vi "1 - 测试机台交互.vi"(6 "测试机台选择":tag="VB8012-30F490B", 7 "Error In":errorcluster caption="Error In (no error)", 8 "逻辑分析仪参数输入":T2, 9 "可编程电源参数输入":T3, 10 "显示控件引用输入":T1) -> (0 "error out":errorcluster caption="错误输出", 2 "采集信号输出":waveform(dbl)[](array[waveform]), 3 "显示控件引用输出":T1)   [LabVIEW 2019]
uses:
  <vilib>/VirtualBench/_PS Configure Voltage Output0.vi
  <vilib>/VirtualBench/_FGEN Configure Standard Waveform0.vi
  <vilib>/VirtualBench/_MSO Configure Timing0.vi
  <vilib>/VirtualBench/_MSO Configure Digital Edge Trigger0.vi
  <vilib>/VirtualBench/_MSO Configure Analog Edge Trigger0.vi
  <vilib>/VirtualBench/_MSO Configure Digital Pattern Trigger0.vi
  <vilib>/VirtualBench/VirtualBench.lvlib
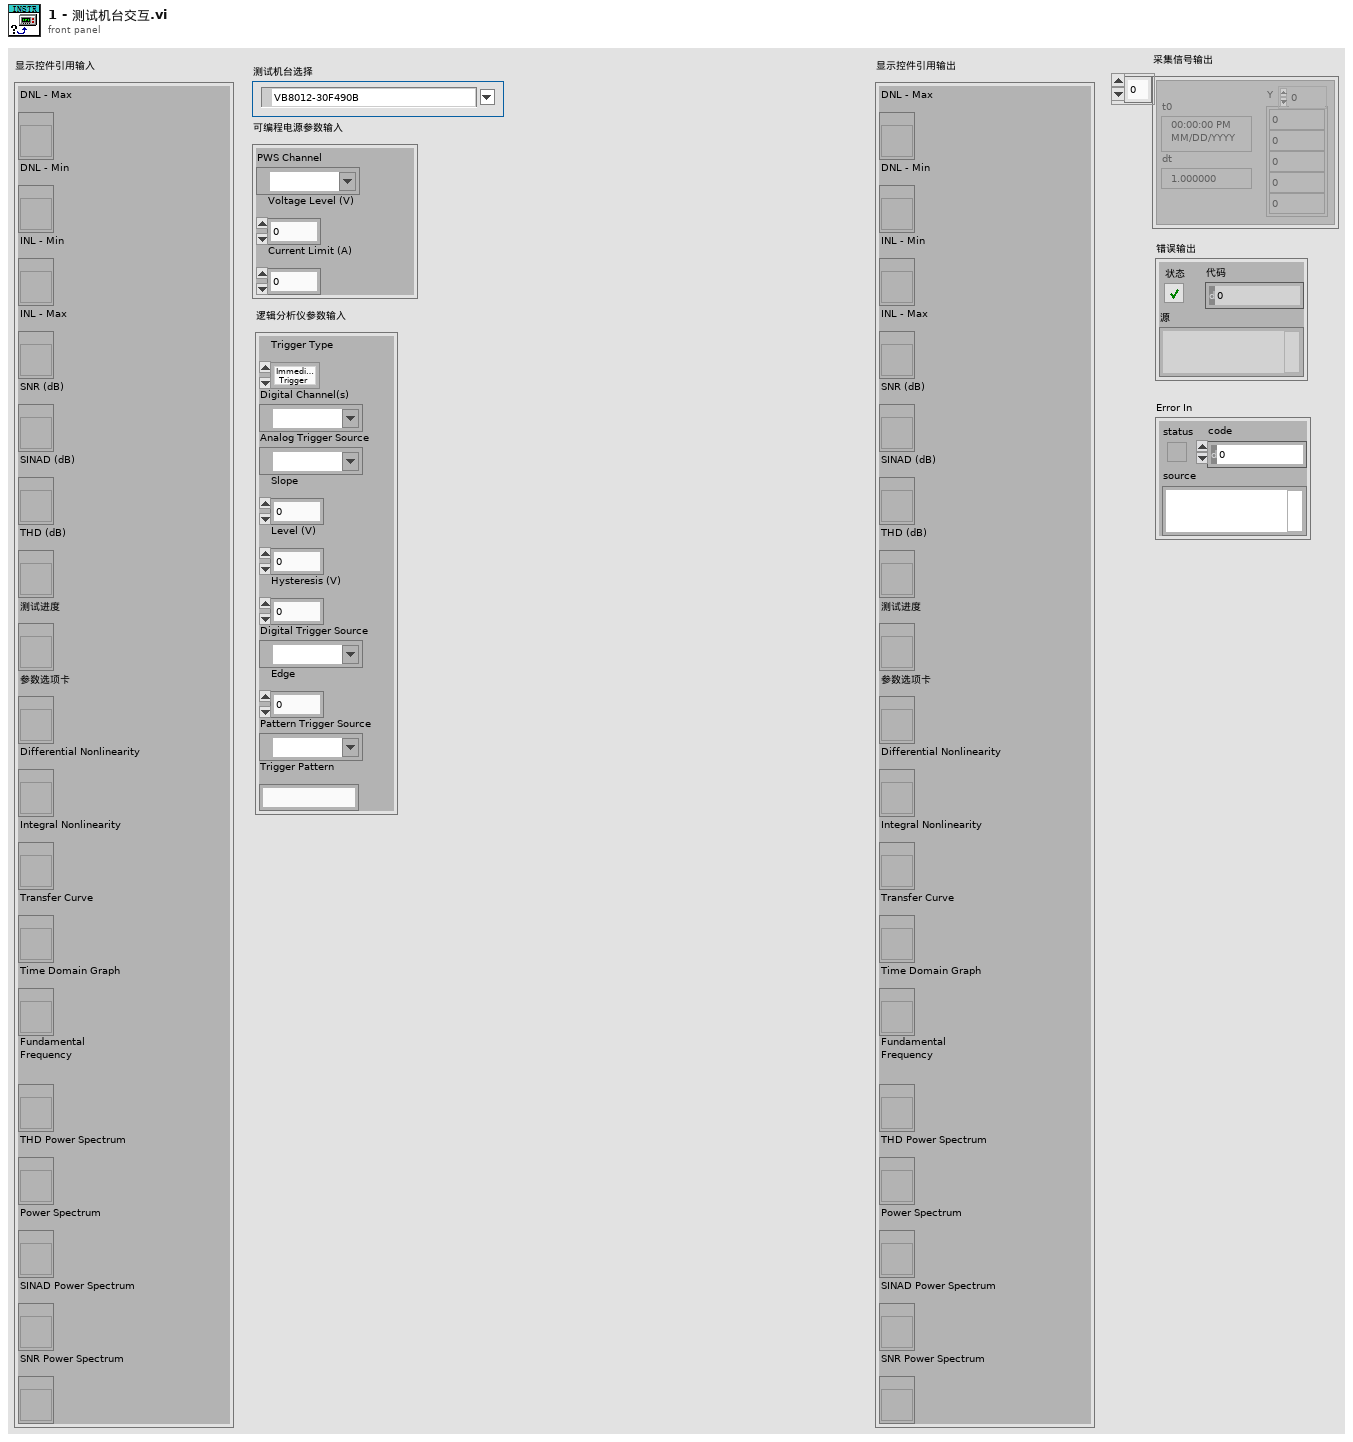
[diagram p1: front panel]
types:
  T1 = cluster{"DNL - Max":refnum<vi>, "DNL - Min":refnum<vi>, "INL - Min":refnum<vi>, "INL - Max":refnum<vi>, "SNR (dB)":refnum<vi>, "SINAD (dB)":refnum<vi>, "THD (dB)":refnum<vi>, "测试进度":refnum<vi>, "参数选项卡":refnum<vi>, "Differential Nonlinearity":refnum<vi>, "Integral Nonlinearity":refnum<vi>, "Transfer Curve":refnum<vi>, "Time Domain Graph":refnum<vi>, "Fundamental\nFrequency":refnum<vi>, "THD Power Spectrum":refnum<vi>, "Power Spectrum":refnum<vi>, "SINAD Power Spectrum":refnum<vi>, "SNR Power Spectrum":refnum<vi>}
  T2 = cluster{"Trigger Type":enum32{"Immediate Trigger", "Digital Trigger", "Analog Trigger", "Pattern Trigger"}, "Digital Channel(s)":tag, "Analog Trigger Source":tag, "Slope":i32, "Level (V)":dbl, "Hysteresis (V)":dbl, "Digital Trigger Source":tag, "Edge":i32, "Pattern Trigger Source":tag, "Trigger Pattern":string}
  T3 = cluster{"PWS Channel":tag, "Voltage Level (V)":dbl, "Current Limit (A)":dbl}
  T4 = enum32{"Time Domain", "Power Spectrum", "THD", "SINAD", "SNR", "DNL", "INL", "Transfer Curve"}
  T5 = enum32{"Immediate Trigger", "Digital Trigger", "Analog Trigger", "Pattern Trigger"}
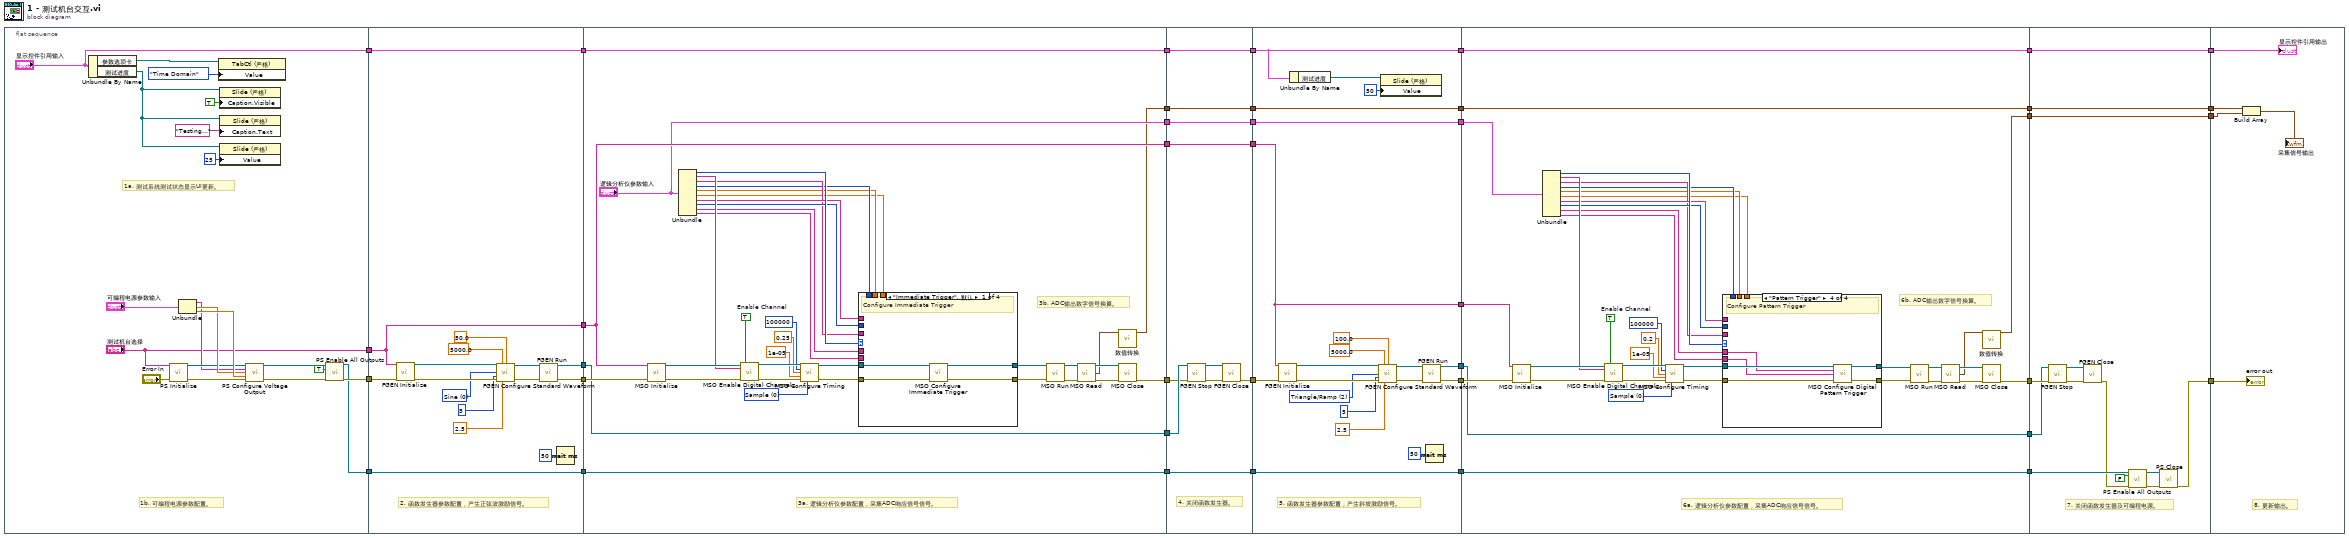
[diagram p0: block diagram]
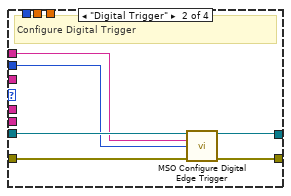
[diagram p2: hidden frame]
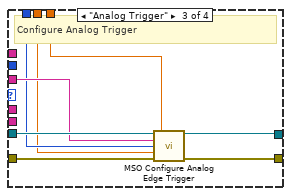
[diagram p3: hidden frame]
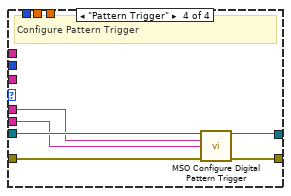
[diagram p4: hidden frame]
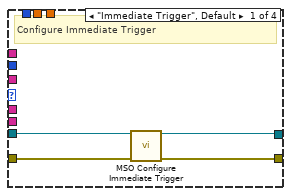
[diagram p5: hidden frame]
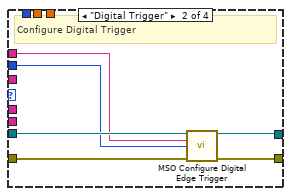
[diagram p6: hidden frame]
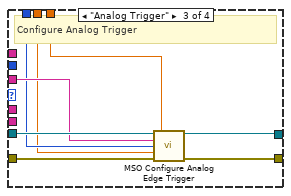
[diagram p7: hidden frame]
diagram:
  n1 = flat-sequence {
    tunnel: [w50] -> w39
    tunnel: ["测试机台选择"] -> w38
    tunnel: ["显示控件引用输入"] -> w8
    tunnel: [w49] -> w6
    tunnel: w39 -> [w71]
    tunnel: w38 -> [w63]
    tunnel: [w65] -> w37
    tunnel: [w64] -> w36
    tunnel: [w63] -> w35
    tunnel: [w62] -> w9
    tunnel: w8 -> [w62]
    tunnel: w6 -> [w61]
    tunnel: [w61] -> w1
    tunnel: w37 -> [w82]
    tunnel: w36 -> [w99]
    tunnel: w35 -> [w80]
    tunnel: [w82] -> w34
    tunnel: [w81] -> w33
    tunnel: [w80] -> w30
    tunnel: ["逻辑分析仪参数输入"] -> w25
    tunnel: [w78] -> w21
    tunnel: [w77] -> w10
    tunnel: w9 -> [w77]
    tunnel: [w76] -> w2
    tunnel: w1 -> [w76]
    tunnel: w34 -> [w144]
    tunnel: w33 -> [w143]
    tunnel: [w141] -> w32
    tunnel: [w140] -> w31
    tunnel: w30 -> [w140]
    tunnel: [w139] -> w26
    tunnel: w25 -> [w139]
    tunnel: w21 -> [w138]
    tunnel: [w138] -> w18
    tunnel: [w137] -> w11
    tunnel: w10 -> [w137]
    tunnel: [w136] -> w3
    tunnel: w2 -> [w136]
    tunnel: w32 -> [w156]
    tunnel: w31 -> [w153]
    tunnel: [w155] -> w29
    tunnel: [w154] -> w28
    tunnel: [w153] -> w27
    tunnel: w26 -> [w152]
    tunnel: [w152] -> w24
    tunnel: [w151] -> w19
    tunnel: w18 -> [w151]
    tunnel: [w146] -> w12
    tunnel: w11 -> [w146]
    tunnel: [w150] -> w4
    tunnel: w3 -> [w150]
    tunnel: w29 -> [w175]
    tunnel: w28 -> [w171]
    tunnel: w27 -> [w174]
    tunnel: w24 -> [w173]
    tunnel: [w172] -> w23
    tunnel: [w171] -> w22
    tunnel: [w170] -> w20
    tunnel: w19 -> [w170]
    tunnel: [w167] -> w17
    tunnel: [w169] -> w13
    tunnel: w12 -> [w169]
    tunnel: [w168] -> w5
    tunnel: w4 -> [w168]
    tunnel: w23 -> [w237]
    tunnel: w22 -> [w236]
    tunnel: w20 -> [w235]
    tunnel: w17 -> [w234]
    tunnel: [w235] -> w16
    tunnel: [w234] -> w15
    tunnel: [w233] -> w14
    tunnel: w13 -> [w233]
    tunnel: [w227] -> w7
    tunnel: w5 -> [w229]
    tunnel: w16 -> [w244]
    tunnel: w15 -> [w243]
    tunnel: w14 -> [w240]
    tunnel: w7 -> [w241]
    frame #0 {
      # "1b. 可编程电源参数配置。"
      # "1a. 测试系统测试状态显示UI更新。"
      n2 = Unbundle By Name("显示控件引用输入") -> ("参数选项卡"=w48:refnum<vi>, "测试进度"=w44:refnum<vi>)
      n3 = call <vilib>:"PS Initialize.vi"("Device Name"="测试机台选择", "Error In"="Error In") -> ("Instrument Handle Out"=w56:refnum<k21>, "Error Out"=w52:errorcluster)  [unwired: 12 in]
      n4 = Unbundle("可编程电源参数输入") -> ("PWS Channel"=w55:tag, "Voltage Level (V)"=w57:dbl, "Current Limit (A)"=w58:dbl)
      n5 = property class="TabCtl (严格)"(reference=w48, "Value"=T4."Time Domain" ("值")) -> ()  [unwired: 1 in, 2 out]
      n6 = property class="Slide (严格)"(reference=w44, "Caption.Visible"=TRUE ("标题.可见")) -> ()  [unwired: 1 in, 2 out]
      n7 = property class="Slide (严格)"(reference=w44, "Caption.Text"="Testing..." ("标题.文本")) -> ()  [unwired: 1 in, 2 out]
      n8 = property class="Slide (严格)"(reference=w44, "Value"=u8 25 ("值")) -> ()  [unwired: 1 in, 2 out]
      n9 = call-poly <vilib>:"PS Configure Voltage Output.vi"("Instrument Handle In"=w56, "Channel"=w55, "Voltage Level"=w57, "Current Limit"=w58, "Error In"=w52) -> ("Instrument Handle Out"=w59:refnum<k21>, "Error Out"=w53:errorcluster)  [unwired: 9 in]
      n10 = call <vilib>:"PS Enable All Outputs.vi"("Instrument Handle In"=w59, "Enable Outputs"=TRUE ("Enable Output"), "Error In"=w53) -> ("Instrument Handle Out"=w49:refnum<k21>, "Error Out"=w50:errorcluster)  [unwired: 11 in]
    }
    frame #1 {
      w68 = 0 items=["Sine", "Square", "Triangle/Ramp", "DC"] ("Waveform Function")
      # "2. 函数发生器参数配置，产生正弦波激励信号。"
      n11 = call <vilib>:"FGEN Initialize.vi"("Device Name"=w63, "Error In"=w71) -> ("Instrument Handle Out"=w72:refnum<k21>, "Error Out"=w73:errorcluster)  [unwired: 12 in]
      n12 = call-poly <vilib>:"FGEN Configure Standard Waveform.vi"("Instrument Handle In"=w72, "Frequency"=5000.0 ("Frequency (Hz)"), "Duty Cycle"=50.0, "Waveform Function"=w68, "Amplitude"=5 ("Amplitude (V)"), "Error In"=w73, "DC Offset"=2.5 ("DC Offset (V)")) -> ("Instrument Handle Out"=w74:refnum<k21>, "Error Out"=w75:errorcluster)  [unwired: 7 in]
      n13 = call <vilib>:"FGEN Run.vi"("Instrument Handle In"=w74, "Error In"=w75) -> ("Instrument Handle Out"=w65:refnum<k21>, "Error Out"=w64:errorcluster)  [unwired: 12 in]
      n14 = Wait (ms)(milliseconds to wait=u32 50 ("等待时间（毫秒）")) -> ()  [unwired: 1 out]
    }
    frame #2 {
      w106 = TRUE  # Enable Channel
      w111 = 0 items=["Sample", "Peak Detect"] ("Sampling Mode")
      # "3b. ADC输出数字信号换算。"
      # "3a. 逻辑分析仪参数配置，采集ADC响应信号信号。"
      n15 = call <vilib>:"MSO Initialize.vi"("Device Name"=w80, "Error In"=w99) -> ("Instrument Handle Out"=w103:refnum<k21>, "Error Out"=w102:errorcluster)  [unwired: 12 in]
      n16 = Unbundle("逻辑分析仪参数输入") -> ("Trigger Type"=w94:T5, "Digital Channel(s)"=w98:tag, "Analog Trigger Source"=w91:tag, "Slope"=w90:i32, "Level (V)"=w89:dbl, "Hysteresis (V)"=w88:dbl, "Digital Trigger Source"=w93:tag, "Edge"=w92:i32, "Pattern Trigger Source"=w87:tag, "Trigger Pattern"=w86:string)
      n17 = call <vilib>:"MSO Enable Digital Channels.vi"("Instrument Handle In"=w103, "Enable Channel"=w106, "Channel"=w98, "Error In"=w102) -> ("Instrument Handle Out"=w107:refnum<k21>, "Error Out"=w108:errorcluster)  [unwired: 10 in]
      n18 = call-poly <vilib>:"MSO Configure Timing.vi"("Instrument Handle In"=w107, "Sample Rate"=100000 ("Sample Rate (Hz)"), "Acquisition Time (s)"=0.25, "Pretrigger Time (s)"=1e-05, "Error In"=w108, "Sampling Mode"=w111) -> ("Instrument Handle Out"=w110:refnum<k21>, "Error Out"=w109:errorcluster)  [unwired: 8 in]
      n19 = case shown="\"Immediate Trigger\", 默认" w94 {
        tunnel: w110 -> [w115 w119 w126 w133]
        tunnel: w109 -> [w113 w120 w129 w132]
        tunnel: [w114 w118 w127 w134] -> w101
        tunnel: [w112 w121 w128 w135] -> w100
        tunnel: w93 -> [_ w117 _ _]
        tunnel: w92 -> [_ w116 _ _]
        tunnel: w91 -> [_ _ w125 _]
        tunnel: w90 -> [_ _ w124 _]
        tunnel: w89 -> [_ _ w123 _]
        tunnel: w88 -> [_ _ w122 _]
        tunnel: w87 -> [_ _ _ w131]
        tunnel: w86 -> [_ _ _ w130]
        frame "Immediate Trigger", Default {
          # "Configure Immediate Trigger"
          n20 = call <vilib>:"MSO Configure Immediate Trigger.vi"("Instrument Handle In"=w115, "Error In"=w113) -> ("Instrument Handle Out"=w114:refnum<k21>, "Error Out"=w112:errorcluster)  [unwired: 12 in]
        }
        frame "Digital Trigger" {
          # "Configure Digital Trigger"
          n21 = call-poly <vilib>:"MSO Configure Digital Edge Trigger.vi"("Instrument Handle In"=w119, "Trigger Source"=w117, "Trigger Slope"=w116, "Error In"=w120) -> ("Instrument Handle Out"=w118:refnum<k21>, "Error Out"=w121:errorcluster)  [unwired: 10 in]
        }
        frame "Analog Trigger" {
          # "Configure Analog Trigger"
          n22 = call-poly <vilib>:"MSO Configure Analog Edge Trigger.vi"("Instrument Handle In"=w126, "Trigger Hysteresis"=w122, "Trigger Source"=w125, "Trigger Slope"=w124, "Trigger Level"=w123, "Error In"=w129) -> ("Instrument Handle Out"=w127:refnum<k21>, "Error Out"=w128:errorcluster)  [unwired: 8 in]
        }
        frame "Pattern Trigger" {
          # "Configure Pattern Trigger"
          n23 = call-poly <vilib>:"MSO Configure Digital Pattern Trigger.vi"("Instrument Handle In"=w133, "Trigger Source"=w131, "Trigger Pattern"=w130, "Error In"=w132) -> ("Instrument Handle Out"=w134:refnum<k21>, "Error Out"=w135:errorcluster)  [unwired: 10 in]
        }
      }
      n24 = call <vilib>:"MSO Run.vi"("Instrument Handle In"=w101, "Error In"=w100) -> ("Instrument Handle Out"=w105:refnum<k21>, "Error Out"=w104:errorcluster)  [unwired: 12 in]
      n25 = call <vilib>:"MSO Read.vi"("Instrument Handle In"=w105, "Error In"=w104) -> ("Instrument Handle Out"=w84:refnum<k21>, "Digital Waveform"=w83:digitalwaveform, "Error Out"=w85:errorcluster)  [unwired: 8 in, 3 out]
      n26 = call "数值转换.vi"("Digital Waveform"=w83) -> ("Waveform"=w78:waveform(dbl))  [unwired: 9 in, 1 out]
      n27 = call <vilib>:"MSO Close.vi"("Instrument Handle In"=w84, "Error In"=w85) -> ("Error Out"=w81:errorcluster)  [unwired: 13 in]
    }
    frame #3 {
      # "4. 关闭函数发生器。"
      n28 = call <vilib>:"FGEN Stop.vi"("Instrument Handle In"=w144, "Error In"=w143) -> ("Instrument Handle Out"=w142:refnum<k21>, "Error Out"=w145:errorcluster)  [unwired: 12 in]
      n29 = call <vilib>:"FGEN Close.vi"("Instrument Handle In"=w142, "Error In"=w145) -> ("Error Out"=w141:errorcluster)  [unwired: 13 in]
    }
    frame #4 {
      w159 = 2 items=["Sine", "Square", "Triangle/Ramp", "DC"] ("Waveform Function")
      # "5. 函数发生器参数配置，产生斜坡激励信号。"
      n30 = call <vilib>:"FGEN Initialize.vi"("Device Name"=w153, "Error In"=w156) -> ("Instrument Handle Out"=w162:refnum<k21>, "Error Out"=w163:errorcluster)  [unwired: 12 in]
      n31 = Unbundle By Name(w146) -> ("测试进度"=w148:refnum<vi>)
      n32 = call-poly <vilib>:"FGEN Configure Standard Waveform.vi"("Instrument Handle In"=w162, "Frequency"=5000.0 ("Frequency (Hz)"), "Duty Cycle"=100.0, "Waveform Function"=w159, "Amplitude"=5 ("Amplitude (V)"), "Error In"=w163, "DC Offset"=2.5 ("DC Offset (V)")) -> ("Instrument Handle Out"=w164:refnum<k21>, "Error Out"=w165:errorcluster)  [unwired: 7 in]
      n33 = property class="Slide (严格)"(reference=w148, "Value"=u8 50 ("值")) -> ()  [unwired: 1 in, 2 out]
      n34 = call <vilib>:"FGEN Run.vi"("Instrument Handle In"=w164, "Error In"=w165) -> ("Instrument Handle Out"=w154:refnum<k21>, "Error Out"=w155:errorcluster)  [unwired: 12 in]
      n35 = Wait (ms)(milliseconds to wait=u32 50 ("等待时间（毫秒）")) -> ()  [unwired: 1 out]
    }
    frame #5 {
      w197 = TRUE  # Enable Channel
      w202 = 0 items=["Sample", "Peak Detect"] ("Sampling Mode")
      # "6b. ADC输出数字信号换算。"
      # "6a. 逻辑分析仪参数配置，采集ADC响应信号信号。"
      n36 = call <vilib>:"MSO Initialize.vi"("Device Name"=w174, "Error In"=w175) -> ("Instrument Handle Out"=w194:refnum<k21>, "Error Out"=w193:errorcluster)  [unwired: 12 in]
      n37 = Unbundle(w173) -> ("Trigger Type"=w186:T5, "Digital Channel(s)"=w190:tag, "Analog Trigger Source"=w183:tag, "Slope"=w182:i32, "Level (V)"=w181:dbl, "Hysteresis (V)"=w180:dbl, "Digital Trigger Source"=w185:tag, "Edge"=w184:i32, "Pattern Trigger Source"=w179:tag, "Trigger Pattern"=w178:string)
      n38 = call <vilib>:"MSO Enable Digital Channels.vi"("Instrument Handle In"=w194, "Enable Channel"=w197, "Channel"=w190, "Error In"=w193) -> ("Instrument Handle Out"=w198:refnum<k21>, "Error Out"=w199:errorcluster)  [unwired: 10 in]
      n39 = call-poly <vilib>:"MSO Configure Timing.vi"("Instrument Handle In"=w198, "Sample Rate"=100000 ("Sample Rate (Hz)"), "Acquisition Time (s)"=0.2, "Pretrigger Time (s)"=1e-05, "Error In"=w199, "Sampling Mode"=w202) -> ("Instrument Handle Out"=w201:refnum<k21>, "Error Out"=w200:errorcluster)  [unwired: 8 in]
      n40 = case shown="\"Pattern Trigger\"" w186 {
        tunnel: w201 -> [w206 w210 w217 w224]
        tunnel: w200 -> [w204 w211 w220 w223]
        tunnel: [w205 w209 w218 w225] -> w192
        tunnel: [w203 w212 w219 w226] -> w191
        tunnel: w185 -> [_ w208 _ _]
        tunnel: w184 -> [_ w207 _ _]
        tunnel: w183 -> [_ _ w216 _]
        tunnel: w182 -> [_ _ w215 _]
        tunnel: w181 -> [_ _ w214 _]
        tunnel: w180 -> [_ _ w213 _]
        tunnel: w179 -> [_ _ _ w222]
        tunnel: w178 -> [_ _ _ w221]
        frame "Immediate Trigger", Default {
          # "Configure Immediate Trigger"
          n41 = call <vilib>:"MSO Configure Immediate Trigger.vi"("Instrument Handle In"=w206, "Error In"=w204) -> ("Instrument Handle Out"=w205:refnum<k21>, "Error Out"=w203:errorcluster)  [unwired: 12 in]
        }
        frame "Digital Trigger" {
          # "Configure Digital Trigger"
          n42 = call-poly <vilib>:"MSO Configure Digital Edge Trigger.vi"("Instrument Handle In"=w210, "Trigger Source"=w208, "Trigger Slope"=w207, "Error In"=w211) -> ("Instrument Handle Out"=w209:refnum<k21>, "Error Out"=w212:errorcluster)  [unwired: 10 in]
        }
        frame "Analog Trigger" {
          # "Configure Analog Trigger"
          n43 = call-poly <vilib>:"MSO Configure Analog Edge Trigger.vi"("Instrument Handle In"=w217, "Trigger Hysteresis"=w213, "Trigger Source"=w216, "Trigger Slope"=w215, "Trigger Level"=w214, "Error In"=w220) -> ("Instrument Handle Out"=w218:refnum<k21>, "Error Out"=w219:errorcluster)  [unwired: 8 in]
        }
        frame "Pattern Trigger" {
          # "Configure Pattern Trigger"
          n44 = call-poly <vilib>:"MSO Configure Digital Pattern Trigger.vi"("Instrument Handle In"=w224, "Trigger Source"=w222, "Trigger Pattern"=w221, "Error In"=w223) -> ("Instrument Handle Out"=w225:refnum<k21>, "Error Out"=w226:errorcluster)  [unwired: 10 in]
        }
      }
      n45 = call <vilib>:"MSO Run.vi"("Instrument Handle In"=w192, "Error In"=w191) -> ("Instrument Handle Out"=w196:refnum<k21>, "Error Out"=w195:errorcluster)  [unwired: 12 in]
      n46 = call <vilib>:"MSO Read.vi"("Instrument Handle In"=w196, "Error In"=w195) -> ("Instrument Handle Out"=w176:refnum<k21>, "Digital Waveform"=w166:digitalwaveform, "Error Out"=w177:errorcluster)  [unwired: 8 in, 3 out]
      n47 = call "数值转换.vi"("Digital Waveform"=w166) -> ("Waveform"=w167:waveform(dbl))  [unwired: 9 in, 1 out]
      n48 = call <vilib>:"MSO Close.vi"("Instrument Handle In"=w176, "Error In"=w177) -> ("Error Out"=w172:errorcluster)  [unwired: 13 in]
    }
    frame #6 {
      # "7. 关闭函数发生器及可编程电源。"
      n49 = call <vilib>:"FGEN Stop.vi"("Instrument Handle In"=w236, "Error In"=w237) -> ("Instrument Handle Out"=w239:refnum<k21>, "Error Out"=w238:errorcluster)  [unwired: 12 in]
      n50 = call <vilib>:"FGEN Close.vi"("Instrument Handle In"=w239, "Error In"=w238) -> ("Error Out"=w228:errorcluster)  [unwired: 13 in]
      n51 = call <vilib>:"PS Enable All Outputs.vi"("Instrument Handle In"=w229, "Enable Outputs"=FALSE ("Enable Output"), "Error In"=w228) -> ("Instrument Handle Out"=w232:refnum<k21>, "Error Out"=w231:errorcluster)  [unwired: 11 in]
      n52 = call <vilib>:"PS Close.vi"("Instrument Handle In"=w232, "Error In"=w231) -> ("Error Out"=w227:errorcluster)  [unwired: 13 in]
    }
    frame #7 {
      # "8. 更新输出。"
      n53 = Build Array(w244, w243) -> (→"采集信号输出":waveform(dbl)[])
      "error out" <- w241
      "显示控件引用输出" <- w240
    }
  }
